vi "sv_One Harmonic Notch Filter.vi"(8 "error in (no error)":errorcluster, 9 "bandwidth [order]":dbl=1.0 format="%0.2f", 10 "specific harmonic":dbl=1.0 format="%0.2f", 11 "fs":dbl=10.0) -> (0 "error out":errorcluster, 2 "delay [samples]":i32, 3 "FIR filter":dbl[](array[numeric]))   [LabVIEW 2017, in "SoundVib_ContSweptSine.lvlib"]
uses:
  <vilib>/addons/Sound and Vibration/svt_Continuous Swept Sine/SoundVib_ContSweptSine.lvlib
  <vilib>/addons/Sound and Vibration/svt_Continuous Swept Sine/subVIs/sv_Continuous Swept-Sine Errors.ctl
  <vilib>/Analysis/1siggen.llb/Ramp Pattern by Samples.vi
  <vilib>/addons/Sound and Vibration/Order Analysis/Resample Order Tracking/SoundVib_Resampling.lvlib
  <vilib>/Analysis/NI_AALBase.lvlib
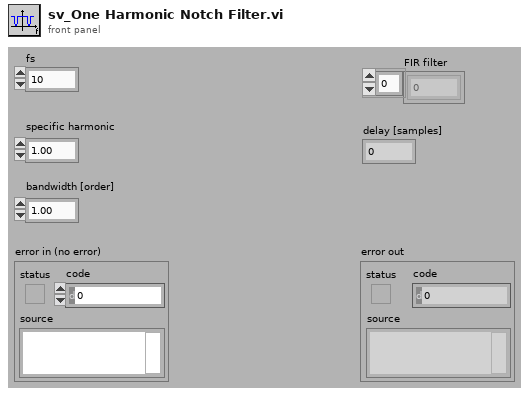
[diagram p1: front panel]
types:
  T1 = typedef "SoundVib_ContSweptSine.lvlib/sv_Continuous Swept-Sine Errors.ctl" = enum16{"Invalid AI sampling rate", "Item not found", "Invalid initial phase"}
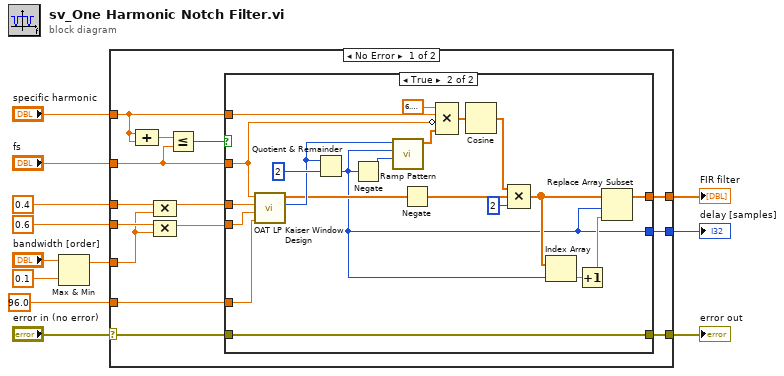
[diagram p0: block diagram]
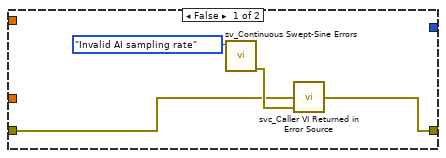
[diagram p2: hidden frame]
diagram:
  n1 = Max & Min(x="bandwidth [order]", y=0.1) -> (max(x,y)=w1:dbl)  [unwired: 1 out]
  n2 = case shown="No Error" "error in (no error)" {
    selector: "error in (no error)" -> [w20 w52]
    tunnel: 0.4 ("passband") -> [w26 _]
    tunnel: 0.6 ("stopband") -> [w25 _]
    tunnel: 96.0 ("A stop [dB]") -> [w24 _]
    tunnel: [w23 _] -> w9
    tunnel: [w22 _] -> w8
    tunnel: "fs" -> [w16 _]
    tunnel: "specific harmonic" -> [w18 _]
    tunnel: [w19 w52] -> w4
    tunnel: w1 -> [w13 _]
    frame No Error {
      n3 = Compound Arithmetic op=ADD(w18, w18) -> (w17:dbl)
      n4 = Compound Arithmetic op=MULTIPLY(w26, w13) -> (w15:dbl)
      n5 = Compound Arithmetic op=MULTIPLY(w25, w13) -> (w14:dbl)
      n6 = Less Or Equal?(x=w17, y=w16) -> (x <= y?=w21:bool)
      n7 = case shown="True" w21 {
        tunnel: w15 -> [_ w51]
        tunnel: w14 -> [_ w50]
        tunnel: w24 -> [_ w49]
        tunnel: [_ w31] -> w23
        tunnel: [_ w33] -> w22
        tunnel: w16 -> [_ w39]
        tunnel: w18 -> [_ w38]
        tunnel: w20 -> [w27 w37]
        tunnel: [w29 w37] -> w19
        frame False {
          n8 = call <vilib>:"sv_Continuous Swept-Sine Errors.vi"("continuous swept-sine error"=sv_Continuous_Swept-Sine_Errors."Invalid AI sampling rate") -> ("error out"=w28:errorcluster)  [unwired: 10 in]
          n9 = call <vilib>:"svc_Caller VI Returned in Error Source.vi"("warning input to caller"=w28, "error in (no error)"=w27) -> ("error out"=w29:errorcluster)  [unwired: 3 in]
        }
        frame True {
          n10 = call <vilib>:"OAT LP Kaiser Window Design.vi"("A stop [dB]"=w49, "stopband"=w50, "passband"=w51, "fs"=w39) -> ("taps"=w47:i32, "filter coefficients"=w41:dbl[])  [unwired: 5 in, 1 out]
          n11 = Quotient & Remainder(x=w47, y=2) -> (floor(x/y)=w31:i32)  [unwired: 1 out]
          n12 = Negate(x=w31) -> (-x=w46:i32)
          n13 = call-poly <vilib>:"Ramp Pattern.vi"("start"=w46, "end"=w31, "samples"=w47) -> ("Ramp Pattern"=w45:dbl[])  [unwired: 7 in, 1 out]
          n14 = Negate(x=w41) -> (-x=w35:dbl[])
          n15 = Compound Arithmetic op=MULTIPLY(6.283185307179586, w38, invert w39, w45) -> (w43:dbl[])
          n16 = Cosine(x=w43) -> (cos(x)=w42:dbl[])
          n17 = Compound Arithmetic op=MULTIPLY(w42, w35, 2) -> (w36:dbl[])
          n18 = Index Array(array=w36, index=w31) -> (element=w34:dbl)
          n19 = Increment(x=w34) -> (x+1=w32:dbl)
          n20 = Replace Array Subset(array=w36, new element=w32, index=w31) -> (w33:dbl[])
        }
      }
    }
    frame Error {
    }
  }
  "delay [samples]" <- w9
  "FIR filter" <- w8
  "error out" <- w4
